vi "COMI Last Error.vi"() -> (3 "function return":i32)   [LabVIEW 2017, in "Comidll.lvlib"]
doc: "int (COMI_LastError) (void);"
uses:
  <userlib>/Comidll/Comidll.lvlib
  <userlib>/Comidll/Comidll.dll
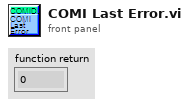
[diagram p1: front panel]
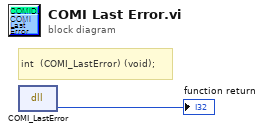
[diagram p0: block diagram]
diagram:
  # "int\t\t(COMI_LastError) (void);"
  n1 = dll-call lib="C:/Program Files/National Instruments/LabVIEW 2017/user.lib/Comidll/Comidll.*" fn="COMI_LastError"() -> (→"function return":i32)  [unwired: 3 in, 2 out]
